vi "File Progress Global.vi"() -> ()   [LabVIEW 2016]
panel:
  in  "Stop":bool
  in  "File Progress Cluster":cluster{"Channel Count":i32, "Offset Count":i64}
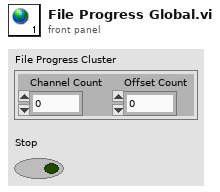
[diagram p1: front panel]
diagram:
